vi "OutputTest1.vi"() -> ()   [LabVIEW 2011]
panel:
  out "DEC Error":errorcluster
  in  "Telescope Slewing ?":bool
  in  "RA Period":i32=10 min=10 max=1000 step=1
  out "RA Error":errorcluster
  out "P2.6":bool
  out "P2.7":bool
  in  "stop":bool
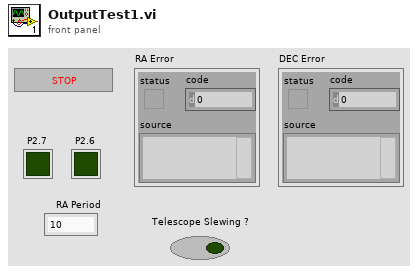
[diagram p1: front panel]
types:
  T1 = cluster{"North Task":refnum<k21>, "South Task":refnum<k21>, "East Task":refnum<k21>, "West Task":refnum<k21>}
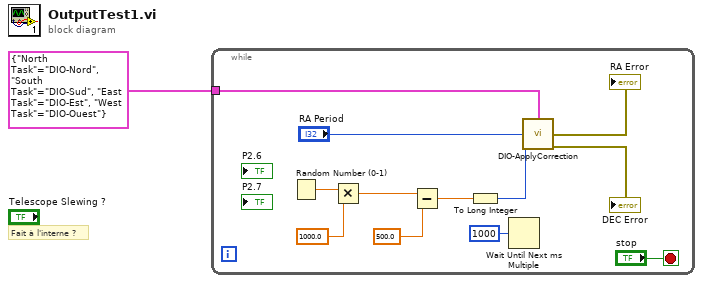
[diagram p0: block diagram]
diagram:
  # "Fait à l'interne ?"
  n1 = while {
    tunnel: T1 {"North Task"="DIO-Nord", "South Task"="DIO-Sud", "East Task"="DIO-Est", "West Task"="DIO-Ouest"} ("TaskCluster") -> [w12]
    stop <- "stop" stop-if-true
    n2 = Random Number (0-1)() -> (number: 0 to 1=w8:dbl)
    n3 = Multiply(x=w8, y=1000.0) -> (x*y=w3:dbl)
    n4 = Subtract(x=w3, y=500.0) -> (x-y=w6:dbl)
    n5 = To Long Integer(number=w6) -> (32bit integer=w2:i32)
    n6 = Wait Until Next ms Multiple(millisecond multiple=u32 1000) -> ()  [unwired: 1 out]
    n7 = call "DIO-ApplyCorrection.vi"("TaskCluster"=w12, "NordSud(ms)"="RA Period", "EstOuest(ms)"=w2) -> ("GuiderRA Error"=→"RA Error":errorcluster, "GuiderDEC Error"=→"DEC Error":errorcluster)  [unwired: 11 in]
  }
